vi "rsidr_core_global.vi"() -> ()   [LabVIEW 2020, in "Rohde&Schwarz RTx Oscilloscopes.lvlib"] (continued)
Options"="", "Flags"=0, "Help"="Queries the input capacitance of the probe.\n\nAvailable Repeated Capabilities:\nChannel: CH0, CH1, CH2, CH3, CH4, CHExt\r\n\nRemote-control command(s):\nPROBe<m>:SETup:CAPacitance?"}, {"Level"=2, "Class Only"=FALSE, "Identifier"="RSRTX_ATTR_PROBE_DEGAUSS", "Descriptive Name"="Probe Degauss", "Data Type"=4, "Command"="PROB{Channel}:SET:DEG", "Access"=1, "Range Table"="", "Read Callback"="", "Write Callback"="", "Supported Models"="", "Instrument Options"="", "Flags"=0, "Help"="Demagnetizes the core if it has been magnetized by switching the power on and off, or by an excessive input. Always demagnetize the probe before measurement. The demagnetizing process takes about one second.\n\nAvailable Repeated Capabilities:\nChannel: CH0, CH1, CH2, CH3, CH4, CHExt\r\n\nRemote-control command(s):\nPROBe<m>:SETup:DEGauss"}, {"Level"=2, "Class Only"=FALSE, "Identifier"="RSRTX_ATTR_PROBE_ATTENUATION", "Descriptive Name"="Probe Attenuation", "Data Type"=1, "Command"="PROB{Channel}:SET:ATT?", "Access"=0, "Range Table"="", "Read Callback"="", "Write Callback"="", "Supported Models"="", "Instrument Options"="", "Flags"=0, "Help"="Queries the attenuation of the probe.\n\nAvailable Repeated Capabilities:\nChannel: CH0, CH1, CH2, CH3, CH4, CHExt\r\n\nRemote-control command(s):\nPROBe<m>:SETup:ATTenuation[:AUTO]?"}, {"Level"=2, "Class Only"=FALSE, "Identifier"="RSRTX_ATTR_PROBE_GAIN", "Descriptive Name"="Probe Gain", "Data Type"=1, "Command"="PROB{Channel}:SET:GAIN?", "Access"=0, "Range Table"="RsRtx_rngProbeGain", "Read Callback"="", "Write Callback"="", "Supported Models"="", "Instrument Options"="", "Flags"=0, "Help"="Returns the gain of an automatically detected probe.\n\nAvailable Repeated Capabilities:\nChannel: CH0, CH1, CH2, CH3, CH4, CHExt\r\n\nRemote-control command(s):\nPROBe<m>:SETup:GAIN[:AUTO]?"}, {"Level"=2, "Class Only"=FALSE, "Identifier"="RSRTX_ATTR_PROBE_BANDWIDTH", "Descriptive Name"="Probe Bandwidth", "Data Type"=1, "Command"="PROB{Channel}:SET:BANDwidth?", "Access"=0, "Range Table"="", "Read Callback"="", "Write Callback"="", "Supported Models"="RTM|RTA", "Instrument Options"="", "Flags"=0, "Help"="Queries the bandwidth of the probe.\n\nAvailable Repeated Capabilities:\nChannel: CH0, CH1, CH2, CH3, CH4, CHExt\r\n\nRemote-control command(s):\nPROBe<m>:SETup:BANDwidth?"}, {"Level"=2, "Class Only"=FALSE, "Identifier"="RSRTX_ATTR_PROBE_DC_OFFSET", "Descriptive Name"="Probe DC Offset", "Data Type"=1, "Command"="PROB{Channel}:SET:DCOF?", "Access"=0, "Range Table"="", "Read Callback"="", "Write Callback"="", "Supported Models"="RTM|RTA", "Instrument Options"="", "Flags"=0, "Help"="Retrieves the DC voltage that is measured by the integrated voltmeter of R&S active probes. Switch the voltmeter on before.\n\nAvailable Repeated Capabilities:\nChannel: CH0, CH1, CH2, CH3, CH4, CHExt\r\n\nRemote-control command(s):\nPROBe<m>:SETup:DCOFfset?"}, {"Level"=2, "Class Only"=FALSE, "Identifier"="RSRTX_ATTR_PROBE_CM_OFFSET", "Descriptive Name"="Probe CM Offset", "Data Type"=1, "Command"="PROB{Channel}:SET:CMOF", "Access"=2, "Range Table"="", "Read Callback"="", "Write Callback"="", "Supported Models"="RTM|RTA", "Instrument Options"="", "Flags"=0, "Help"="Configures the CM voltage offset.\n\nAvailable Repeated Capabilities:\nChannel: CH0, CH1, CH2, CH3, CH4, CHExt\r\n\nRemote-control command(s):\nPROBe<m>:SETup:CMOFfset"}, {"Level"=2, "Class Only"=FALSE, "Identifier"="RSRTX_ATTR_PROBE_ADDITIONAL_OFFSET", "Descriptive Name"="Probe Additional Offset", "Data Type"=1, "Command"="PROB{Channel}:SET:UOFF", "Access"=2, "Range Table"="", "Read Callback"="", "Write Callback"="", "Supported Models"="RTM|RTA", "Instrument Options"="", "Flags"=0, "Help"="Sets an additional probe offset.\n\nAvailable Repeated Capabilities:\nChannel: CH0, CH1, CH2, CH3, CH4, CHExt\r\n\nRemote-control command(s):\nPROBe<m>:SETup:UOFFset"}, {"Level"=2, "Class Only"=FALSE, "Identifier"="RSRTX_ATTR_PROBE_VOLTMETER_ENABLED", "Descriptive Name"="Probe Voltmeter Enabled", "Data Type"=3, "Command"="PROB{Channel}:SET:OFFS", "Access"=2, "Range Table"="", "Read Callback"="", "Write Callback"="", "Supported Models"="RTM|RTA", "Instrument Options"="", "Flags"=0, "Help"="Switches the integrated voltmeter of an R&S active probe on or off.\n\nAvailable Repeated Capabilities:\nChannel: CH0, CH1, CH2, CH3, CH4, CHExt\r\n\nRemote-control command(s):\nPROBe<m>:SETup:OFFSwitch"}, {"Level"=2, "Class Only"=FALSE, "Identifier"="RSRTX_ATTR_PROBE_ATTENUATION_UNIT", "Descriptive Name"="Probe Attenuation Unit", "Data Type"=0, "Command"="PROB{Channel}:SET:ATT:UNIT", "Access"=2, "Range Table"="rsrtx_rngProbeUnit", "Read Callback"="", "Write Callback"="", "Supported Models"="", "Instrument Options"="", "Flags"=0, "Help"="Selects the unit that the probe can measure.\n\nAvailable Repeated Capabilities:\nChannel: CH0, CH1, CH2, CH3, CH4, CHExt\r\n\nRemote-control command(s):\nPROBe<m>:SETup:ATTenuation:UNIT"}, {"Level"=2, "Class Only"=FALSE, "Identifier"="RSRTX_ATTR_PROBE_ATTENUATION_MANUAL", "Descriptive Name"="Probe Attenuation Manual", "Data Type"=1, "Command"="PROB{Channel}:SET:ATT:MAN", "Access"=2, "Range Table"="rsrtx_rngProbeAttenuation", "Read Callback"="", "Write Callback"="", "Supported Models"="", "Instrument Options"="", "Flags"=0, "Help"="Sets the attenuation or gain of the probe if the probe was not detected by the instrument.\n\nAvailable Repeated Capabilities:\nChannel: CH0, CH1, CH2, CH3, CH4, CHExt\r\n\nRemote-control command(s):\nPROBe<m>:SETup:ATTenuation:MANual"}, {"Level"=2, "Class Only"=FALSE, "Identifier"="RSRTX_ATTR_PROBE_GAIN_UNIT", "Descriptive Name"="Probe Gain Unit", "Data Type"=0, "Command"="PROB{Channel}:SET:GAIN:UNIT", "Access"=2, "Range Table"="rsrtx_rngProbeUnit", "Read Callback"="", "Write Callback"="", "Supported Models"="", "Instrument Options"="", "Flags"=0, "Help"="Selects the unit that the probe can measure.\n\nAvailable Repeated Capabilities:\nChannel: CH0, CH1, CH2, CH3, CH4, CHExt\r\n\nRemote-control command(s):\nPROBe<m>:SETup:GAIN:UNIT"}, {"Level"=2, "Class Only"=FALSE, "Identifier"="RSRTX_ATTR_PROBE_GAIN_MANUAL", "Descriptive Name"="Probe Gain Manual", "Data Type"=1, "Command"="PROB{Channel}:SET:GAIN:MAN", "Access"=2, "Range Table"="RsRtx_rngProbeGain", "Read Callback"="", "Write Callback"="", "Supported Models"="", "Instrument Options"="", "Flags"=0, "Help"="Sets the gain of the probe. The gain the the reciprocal of the attenuation (RSRTX_ATTR_PROBE_ATTENUATION_MANUAL).\n\nAvailable Repeated Capabilities:\nChannel: CH0, CH1, CH2, CH3, CH4, CHExt\r\n\nRemote-control command(s):\nPROBe<m>:SETup:GAIN:MANual"}, {"Level"=2, "Class Only"=FALSE, "Identifier"="RSRTX_ATTR_PROBE_MICRO_BUTTON_ACTION", "Descriptive Name"="Probe Micro Button Action", "Data Type"=0, "Command"="PROB{Channel}:SET:MODE", "Access"=2, "Range Table"="rsrtx_rngProbeButtonAction", "Read Callback"="", "Write Callback"="", "Supported Models"="RTM|RTA", "Instrument Options"="", "Flags"=0, "Help"="Select the action that is started with the micro button on the probe head.\n\nAvailable Repeated Capabilities:\nChannel: CH0, CH1, CH2, CH3, CH4, CHExt\r\n\nRemote-control command(s):\nPROBe<m>:SETup:MODE"}, {"Level"=2, "Class Only"=FALSE, "Identifier"="RSRTX_ATTR_PROBE_SOFTWARE_VERSION", "Descriptive Name"="Probe Software Version", "Data Type"=2, "Command"="PROB{Channel}:ID:SWV?", "Access"=0, "Range Table"="", "Read Callback"="", "Write Callback"="", "Supported Models"="RTM|RTA", "Instrument Options"="", "Flags"=0, "Help"="Queries the version of the probe firmware.\n\nAvailable Repeated Capabilities:\nChannel: CH0, CH1, CH2, CH3, CH4, CHExt\r\n\nRemote-control command(s):\nPROBe<m>:ID:SWVersion?"}, {"Level"=2, "Class Only"=FALSE, "Identifier"="RSRTX_ATTR_PROBE_PRODUCTION_DATE", "Descriptive Name"="Probe Production Date", "Data Type"=2, "Command"="PROB{Channel}:ID:PRD?", "Access"=0, "Range Table"="", "Read Callback"="", "Write Callback"="", "Supported Models"="RTM|RTA", "Instrument Options"="", "Flags"=0, "Help"="Queries the production date of the probe.\n\nAvailable Repeated Capabilities:\nChannel: CH0, CH1, CH2, CH3, CH4, CHExt\r\n\nRemote-control command(s):\nPROBe<m>:ID:PRDate?"}, {"Level"=2, "Class Only"=FALSE, "Identifier"="RSRTX_ATTR_PROBE_PART_NUMBER", "Descriptive Name"="Probe Part Number", "Data Type"=2, "Command"="PROB{Channel}:ID:PART?", "Access"=0, "Range Table"="", "Read Callback"="", "Write Callback"="", "Supported Models"="RTM|RTA", "Instrument Options"="", "Flags"=0, "Help"="Queries the R&S part number of the probe.\n\nAvailable Repeated Capabilities:\nChannel: CH0, CH1, CH2, CH3, CH4, CHExt\r\n\nRemote-control command(s):\nPROBe<m>:ID:PARTnumber?"}, {"Level"=2, "Class Only"=FALSE, "Identifier"="RSRTX_ATTR_PROBE_BUILD_NUMBER", "Descriptive Name"="Probe Build Number", "Data Type"=0, "Command"="PROB{Channel}:ID:BUIL?", "Access"=0, "Range Table"="", "Read Callback"="", "Write Callback"="", "Supported Models"="RTM|RTA", "Instrument Options"="", "Flags"=0, "Help"="Queries the build number of the probe software.\n\nAvailable Repeated Capabilities:\nChannel: CH0, CH1, CH2, CH3, CH4, CHExt\r\n\nRemote-control command(s):\nPROBe<m>:ID:BUILd?"}, {"Level"=2, "Class Only"=FALSE, "Identifier"="RSRTX_ATTR_PROBE_SERIAL_NUMBER", "Descriptive Name"="Probe Serial Number", "Data Type"=2, "Command"="PROB{Channel}:ID:SRN?", "Access"=0, "Range Table"="", "Read Callback"="", "Write Callback"="", "Supported Models"="RTM|RTA", "Instrument Options"="", "Flags"=0, "Help"="Queries the serial number of the probe.\n\nAvailable Repeated Capabilities:\nChannel: CH0, CH1, CH2, CH3, CH4, CHExt\r\n\nRemote-control command(s):\nPROBe<m>:ID:SRNumber?"}, {"Level"=2, "Class Only"=FALSE, "Identifier"="RSRTX_ATTR_PROBE_COPY_TO_OFFSET", "Descriptive Name"="Probe Copy To Offset", "Data Type"=4, "Command"="PROB{Channel}:SET:ADV:PMT", "Access"=1, "Range Table"="", "Read Callback"="", "Write Callback"="", "Supported Models"="", "Instrument Options"="", "Flags"=0, "Help"="Sets the measured ProbeMeter&apos;s DC mean value as offset. Make sure that the Probe-Meter is active before you use this attribute.\n\nAvailable Repeated Capabilities:\nChannel: CH0, CH1, CH2, CH3, CH4, CHExt\r\n\nRemote-control command(s):\nPROBe<m>:SETup:ADVanced:PMToffset"}, {"Level"=2, "Class Only"=FALSE, "Identifier"="RSRTX_ATTR_PROBE_ATTENUATOR_RT_ZA15_ENABLED", "Descriptive Name"="Probe Attenuator RT ZA15 Enabled", "Data Type"=3, "Command"="PROB{Channel}:SET:ZAXV", "Access"=2, "Range Table"="", "Read Callback"="", "Write Callback"="", "Supported Models"="", "Instrument Options"="", "Flags"=0, "Help"="Relevant only for differential active probes R&S RT-ZD10, R&S RT-ZD20 or R&S RT-ZD30. If you use the external attenuator R&S RT-ZA15, enable it to include the external attenuation in the measurements.\n\nAvailable Repeated Capabilities:\nChannel: CH0, CH1, CH2, CH3, CH4, CHExt\r\n\nRemote-control command(s):\nPROBe<m>:SETup:ZAXV"}, {"Level"=2, "Class Only"=FALSE, "Identifier"="RSRTX_ATTR_PROBE_ZERO_ADJUST", "Descriptive Name"="Probe Zero Adjust", "Data Type"=1, "Command"="PROB{Channel}:SET:ADV:ZADJ", "Access"=2, "Range Table"="RsRtx_rngProbeZeroAdjust", "Read Callback"="", "Write Callback"="", "Supported Models"="", "Instrument Options"="", "Flags"=0, "Help"="Relevant only for R&S RT-ZCxxB current probes. It sets the waveform to zero position. It corrects the effect of a voltage offset or temperature drift.\n\nAvailable Repeated Capabilities:\nChannel: CH0, CH1, CH2, CH3, CH4, CHExt\r\n\nRemote-control command(s):\nPROBe<m>:SETup:ADVanced:ZADJust"}, {"Level"=2, "Class Only"=FALSE, "Identifier"="RSRTX_ATTR_PROBE_SAVE_ZERO_ADJUST", "Descriptive Name"="Probe Save Zero Adjust", "Data Type"=4, "Command"="PROB{Channel}:SET:ADV:STPR", "Access"=1, "Range Table"="", "Read Callback"="", "Write Callback"="", "Supported Models"="", "Instrument Options"="", "Flags"=0, "Help"="Relevant only for R&S RT-ZCxxB current probes. It saves the zero adjust value in the probe box. If you connect the probe to another channel or to another oscilloscope with Rohde & Schwarz probe interface, the value is read out again.\n\nAvailable Repeated Capabilities:\nChannel: CH0, CH1, CH2, CH3, CH4, CHExt\r\n\nRemote-control command(s):\nPROBe<m>:SETup:ADVanced:STPRobe"}, {"Level"=2, "Class Only"=FALSE, "Identifier"="RSRTX_ATTR_PROBE_INPUT_VOLTAGE_RANGE", "Descriptive Name"="Probe Input Voltage Range", "Data Type"=0, "Command"="PROB{Channel}:SET:ADV:RANG", "Access"=2, "Range Table"="RsRtx_rngProbeInputVoltageRange", "Read Callback"="", "Write Callback"="", "Supported Models"="", "Instrument Options"="", "Flags"=0, "Help"="Relevant for R&S RT-ZHD probes. It sets the voltage range of the probe.\n\nAvailable Repeated Capabilities:\nChannel: CH0, CH1, CH2, CH3, CH4, CHExt\r\n\nRemote-control command(s):\nPROBe<m>:SETup:ADVanced:RANGe"}, {"Level"=2, "Class Only"=FALSE, "Identifier"="RSRTX_ATTR_PROBE_BANDWIDTH_LIMIT", "Descriptive Name"="Probe Bandwidth Limit", "Data Type"=3, "Command"="PROB{Channel}:SET:ADV:FILT", "Access"=2, "Range Table"="", "Read Callback"="", "Write Callback"="", "Supported Models"="", "Instrument Options"="", "Flags"=0, "Help"="Relevant for R&S RT-ZHD probes. It activates the lowpass filter in the probe control box.\n\nAvailable Repeated Capabilities:\nChannel: CH0, CH1, CH2, CH3, CH4, CHExt\r\n\nRemote-control command(s):\nPROBe<m>:SETup:ADVanced:FILTer"}, {"Level"=2, "Class Only"=FALSE, "Identifier"="RSRTX_ATTR_PROBE_AUDIBLE_OVERRANGE", "Descriptive Name"="Probe Audible Overrange", "Data Type"=3, "Command"="PROB{Channel}:SET:ADV:AUD", "Access"=2, "Range Table"="", "Read Callback"="", "Write Callback"="", "Supported Models"="", "Instrument Options"="", "Flags"=0, "Help"="Relevant for R&S RT-ZHD probes. It activates the acoustic overrange warning in the probe control box.\n\nAvailable Repeated Capabilities:\nChannel: CH0, CH1, CH2, CH3, CH4, CHExt\r\n\nRemote-control command(s):\nPROBe<m>:SETup:ADVanced:AUDioverload"}, {"Level"=2, "Class Only"=FALSE, "Identifier"="RSRTX_ATTR_PROBE_MEAS_MODE", "Descriptive Name"="Probe Meas Mode", "Data Type"=0, "Command"="PROB{Channel}:SET:PRM", "Access"=2, "Range Table"="RsRtx_rngProbeMeasMode", "Read Callback"="", "Write Callback"="", "Supported Models"="", "Instrument Options"="", "Flags"=0, "Help"="Relevant only for R&S RT-ZM probes. It sets the measurement mode of modular probes. You can switch between singleended, differential and common mode measurements without reconnecting or resoldering the probe.\n\nAvailable Repeated Capabilities:\nChannel: CH0, CH1, CH2, CH3, CH4, CHExt\r\n\nRemote-control command(s):\nPROBe<m>:SETup:PRMode"}, {"Level"=2, "Class Only"=FALSE, "Identifier"="RSRTX_ATTR_PROBE_AC_COUPLING", "Descriptive Name"="Probe AC Coupling", "Data Type"=3, "Command"="PROB{Channel}:SET:ACC", "Access"=2, "Range Table"="", "Read Callback"="", "Write Callback"="", "Supported Models"="", "Instrument Options"="", "Flags"=0, "Help"="Enables AC coupling in R&S RT-ZPR probes, which removes DC and very low-frequency components. The R&S RT-ZPR probes requires 50   input termination, for which the channel AC coupling is not available. The probe setting allows AC coupling also at 50   inputs.\n\nAvailable Repeated Capabilities:\nChannel: CH0, CH1, CH2, CH3, CH4, CHExt\r\n\nRemote-control command(s):\nPROBe<m>:SETup:ACCoupling"}, {"Level"=2, "Class Only"=TRUE, "Identifier"="", "Descriptive Name"="Probe Meter", "Data Type"=0, "Command"="", "Access"=0, "Range Table"="", "Read Callback"="", "Write Callback"="", "Supported Models"="", "Instrument Options"="", "Flags"=0, "Help"="Shows the measurement result of the integrated R&S ProbeMeter of active Rohde & Schwarz voltage probes.\nIf a single-ended or power rail probe is connected, the ProbeMeter measures DC voltages between the probe tip and ground connection and enables ground-referenced measurements of voltages.\nIf a differential probe is connected, the ProbeMeter measures differential and common\nmode voltages.\nThe ProbeMeter measures continuously and in parallel to the measurements of the oscilloscope. The results are shown below the grid. You can switch off the ProbeMeter using the button below the the results."}, {"Level"=3, "Class Only"=FALSE, "Identifier"="RSRTX_ATTR_PROBE_METER_VISIBILITY", "Descriptive Name"="Probe Meter Visibility", "Data Type"=3, "Command"="PROB{Channel}:PMET:VIS", "Access"=2, "Range Table"="", "Read Callback"="", "Write Callback"="", "Supported Models"="", "Instrument Options"="", "Flags"=0, "Help"="Switches the integrated voltmeter of a Rohde & Schwarz active probe on or off. Only relevant if a Rohde & Schwarz active probe with R&S ProbeMeter is used.\n\nAvailable Repeated Capabilities:\nChannel: CH0, CH1, CH2, CH3, CH4, CHExt\r\n\nRemote-control command(s):\nPROBe<m>:PMETer:VISibility"}, {"Level"=3, "Class Only"=FALSE, "Identifier"="RSRTX_ATTR_PROBE_METER_RESULT_SINGLE", "Descriptive Name"="Probe Meter Result Single", "Data Type"=1, "Command"="PROB{Channel}:PMET:RES:SING?", "Access"=0, "Range Table"="", "Read Callback"="", "Write Callback"="", "Supported Models"="", "Instrument Options"="", "Flags"=0, "Help"="Returns probe meter single result.\n\nAvailable Repeated Capabilities:\nChannel: CH0, CH1, CH2, CH3, CH4, CHExt\r\n\nRemote-control command(s):\nPROBe<m>:PMETer:RESults:SINGle?"}, {"Level"=3, "Class Only"=FALSE, "Identifier"="RSRTX_ATTR_PROBE_METER_RESULT_COMMON", "Descriptive Name"="Probe Meter Result Common", "Data Type"=1, "Command"="PROB{Channel}:PMET:RES:COMM?", "Access"=0, "Range Table"="", "Read Callback"="", "Write Callback"="", "Supported Models"="", "Instrument Options"="", "Flags"=0, "Help"="It returns the common mode voltage, which is the mean voltage between the signal sockets and the ground socket.\n\nAvailable Repeated Capabilities:\nChannel: CH0, CH1, CH2, CH3, CH4, CHExt\r\n\nRemote-control command(s):\nPROBe<m>:PMETer:RESults:COMMon?"}, {"Level"=3, "Class Only"=FALSE, "Identifier"="RSRTX_ATTR_PROBE_METER_RESULT_DIFFERENTIAL", "Descriptive Name"="Probe Meter Result Differential", "Data Type"=1, "Command"="PROB{Channel}:PMET:RES:DIFF?", "Access"=0, "Range Table"="", "Read Callback"="", "Write Callback"="", "Supported Models"="", "Instrument Options"="", "Flags"=0, "Help"="It returns the differential voltage, which is the voltage between the positive and negative signal sockets.\n\nAvailable Repeated Capabilities:\nChannel: CH0, CH1, CH2, CH3, CH4, CHExt\r\n\nRemote-control command(s):\nPROBe<m>:PMETer:RESults:DIFFerential?"}, {"Level"=3, "Class Only"=FALSE, "Identifier"="RSRTX_ATTR_PROBE_METER_RESULT_NEGATIVE", "Descriptive Name"="Probe Meter Result Negative", "Data Type"=1, "Command"="PROB{Channel}:PMET:RES:NEG?", "Access"=0, "Range Table"="", "Read Callback"="", "Write Callback"="", "Supported Models"="", "Instrument Options"="", "Flags"=0, "Help"="It returns the voltage that is measured between the negative signal socket and the ground.\n\nAvailable Repeated Capabilities:\nChannel: CH0, CH1, CH2, CH3, CH4, CHExt\r\n\nRemote-control command(s):\nPROBe<m>:PMETer:RESults:NEGative?"}, {"Level"=3, "Class Only"=FALSE, "Identifier"="RSRTX_ATTR_PROBE_METER_RESULT_POSITIVE", "Descriptive Name"="Probe Meter Result Positive", "Data Type"=1, "Command"="PROB{Channel}:PMET:RES:POS?", "Access"=0, "Range Table"="", "Read Callback"="", "Write Callback"="", "Supported Models"="", "Instrument Options"="", "Flags"=0, "Help"="It returns the voltage that is measured between the positive signal socket and the ground.\n\nAvailable Repeated Capabilities:\nChannel: CH0, CH1, CH2, CH3, CH4, CHExt\r\n\nRemote-control command(s):\nPROBe<m>:PMETer:RESults:POSitive?"}, {"Level"=1, "Class Only"=TRUE, "Identifier"="", "Descriptive Name"="Label", "Data Type"=0, "Command"="", "Access"=0, "Range Table"="", "Read Callback"="", "Write Callback"="", "Supported Models"="", "Instrument Options"="", "Flags"=0, "Help"="The class contains attributes where you can define an additional name label for the selected waveform."}, {"Level"=2, "Class Only"=FALSE, "Identifier"="RSRTX_ATTR_LABEL_ENABLED", "Descriptive Name"="Label Enabled", "Data Type"=3, "Command"="CHAN{Channel}:LAB:STAT", "Access"=2, "Range Table"="", "Read Callback"="", "Write Callback"="", "Supported Models"="", "Instrument Options"="", "Flags"=0, "Help"="Switches the channel name on or off.\n\nAvailable Repeated Capabilities:\nChannel: CH0, CH1, CH2, CH3, CH4, CHExt\r\n\nRemote-control command(s):\nCHANnel<ml>:LABel:STATe"}, {"Level"=2, "Class Only"=FALSE, "Identifier"="RSRTX_ATTR_LABEL_NAME", "Descriptive Name"="Label Name", "Data Type"=2, "Command"="CHAN{Channel}:LAB", "Access"=2, "Range Table"="", "Read Callback"="", "Write Callback"="", "Supported Models"="", "Instrument Options"="", "Flags"=0, "Help"="Specifies a name for the selected channel.\n\nAvailable Repeated Capabilities:\nChannel: CH0, CH1, CH2, CH3, CH4, CHExt\r\n\nRemote-control command(s):\nCHANnel<m>:LABel"}, {"Level"=2, "Class Only"=TRUE, "Identifier"="", "Descriptive Name"="Bus", "Data Type"=0, "Command"="", "Access"=0, "Range Table"="", "Read Callback"="", "Write Callback"="", "Supported Models"="", "Instrument Options"="", "Flags"=0, "Help"="Contain attributes for settings of Bus Label."}, {"Level"=3, "Class Only"=FALSE, "Identifier"="RSRTX_ATTR_BUS_LABEL_ENABLED", "Descriptive Name"="Bus Label Enabled", "Data Type"=3, "Command"="BUS{SerialBus}:LAB:STAT", "Access"=2, "Range Table"="", "Read Callback"="", "Write Callback"="", "Supported Models"="", "Instrument Options"="", "Flags"=0, "Help"="Displays or hides the bus label. The bus label is shown on the the right side of the display.\n\nAvailable Repeated Capabilities:\nSerialBus: SB1, SB2, SB3, SB4\r\n\nRemote-control command(s):\nBUS<b>:LABel:STATe"}, {"Level"=3, "Class Only"=FALSE, "Identifier"="RSRTX_ATTR_BUS_LABEL_NAME", "Descriptive Name"="Bus Label Name", "Data Type"=2, "Command"="BUS{SerialBus}:LAB", "Access"=2, "Range Table"="", "Read Callback"="", "Write Callback"="", "Supported Models"="", "Instrument Options"="", "Flags"=0, "Help"="Defines an additional name label for the selected bus. The maximum name length is 8 characters, and only ASCII characters can be used.\n\nAvailable Repeated Capabilities:\nSerialBus: SB1, SB2, SB3, SB4\r\n\nRemote-control command(s):\nBUS<b>:LABel"}, {"Level"=1, "Class Only"=TRUE, "Identifier"="", "Descriptive Name"="Channel Subsystem", "Data Type"=0, "Command"="", "Access"=0, "Range Table"="", "Read Callback"="", "Write Callback"="", "Supported Models"="", "Instrument Options"="", "Flags"=0, "Help"="Channel-based attributes that you use to configure the channel subsystemof the oscilloscope.  All of the channel subsystem attributes are channel-based."}, {"Level"=2, "Class Only"=FALSE, "Identifier"="RSRTX_ATTR_CHANNEL_ENABLED", "Descriptive Name"="Channel Enabled", "Data Type"=3, "Command"="CHAN{Channel}:STAT", "Access"=2, "Range Table"="", "Read Callback"="", "Write Callback"="", "Supported Models"="", "Instrument Options"="", "Flags"=0, "Help"="Switches the channel signal on or off.\n\nAvailable Repeated Capabilities:\nChannel: CH0, CH1, CH2, CH3, CH4, CHExt\r\n\nRemote-control command(s):\nCHANnel<m>:STATe"}, {"Level"=2, "Class Only"=FALSE, "Identifier"="RSRTX_ATTR_VERTICAL_RANGE", "Descriptive Name"="Vertical Range", "Data Type"=1, "Command"="CHAN{Channel}:RANG", "Access"=2, "Range Table"="", "Read Callback"="", "Write Callback"="", "Supported Models"="", "Instrument Options"="", "Flags"=0, "Help"="Sets the voltage range across the 10 vertical divisions of the diagram.\n\nAvailable Repeated Capabilities:\nChannel: CH0, CH1, CH2, CH3, CH4, CHExt\r\n\nRemote-control command(s):\nCHANnel<m>:RANGe"}, {"Level"=2, "Class Only"=FALSE, "Identifier"="RSRTX_ATTR_VERTICAL_COUPLING", "Descriptive Name"="Vertical Coupling", "Data Type"=0, "Command"="CHAN{Channel}:COUP", "Access"=2, "Range Table"="rsrtx_rngVerticalCoupling", "Read Callback"="", "Write Callback"="", "Supported Models"="", "Instrument Options"="", "Flags"=0, "Help"="Selects the connection of the indicated channel signal.\n\nAvailable Repeated Capabilities:\nChannel: CH0, CH1, CH2, CH3, CH4, CHExt\r\n\nRemote-control command(s):\nCHANnel<m>:COUPling"}, {"Level"=2, "Class Only"=FALSE, "Identifier"="RSRTX_ATTR_VERTICAL_SCALE", "Descriptive Name"="Vertical Scale", "Data Type"=1, "Command"="CHAN{Channel}:SCAL", "Access"=2, "Range Table"="", "Read Callback"="", "Write Callback"="", "Supported Models"="", "Instrument Options"="", "Flags"=0, "Help"="Sets the vertical range per division.\n\nAvailable Repeated Capabilities:\nChannel: CH0, CH1, CH2, CH3, CH4, CHExt\r\n\nRemote-control command(s):\nCHANnel<m>:SCALe"}, {"Level"=2, "Class Only"=FALSE, "Identifier"="RSRTX_ATTR_CHANNEL_OFFSET", "Descriptive Name"="Channel Offset", "Data Type"=1, "Command"="CHAN{Channel}:OFFS", "Access"=2, "Range Table"="", "Read Callback"="", "Write Callback"="", "Supported Models"="", "Instrument Options"="", "Flags"=0, "Help"="The offset voltage is subtracted to correct an offset-affected signal.\n\nAvailable Repeated Capabilities:\nChannel: CH0, CH1, CH2, CH3, CH4, CHExt\r\n\nRemote-control command(s):\nCHANnel<m>:OFFSet"}, {"Level"=2, "Class Only"=FALSE, "Identifier"="RSRTX_ATTR_CHANNEL_ZERO_OFFSET", "Descriptive Name"="Channel Zero Offset", "Data Type"=1, "Command"="CHAN{Channel}:ZOFF", "Access"=2, "Range Table"="", "Read Callback"="", "Write Callback"="", "Supported Models"="", "Instrument Options"="", "Flags"=0, "Help"="Sets the zero offset. Differences in DUT and oscilloscope ground levels may cause larger zero errors affecting the waveform. If the DUT is ground-referenced, the Zero Offset corrects the zero error and sets the probe to the zero level. You can assess the zero error by measuring the mean value of a signal that should return zero.\n\nAvailable Repeated Capabilities:\nChannel: CH0, CH1, CH2, CH3, CH4, CHExt\r\n\nRemote-control command(s):\nCHANnel<m>:ZOFFset[:VALue]"}, {"Level"=2, "Class Only"=FALSE, "Identifier"="RSRTX_ATTR_CHANNEL_BANDWIDTH_LIMIT", "Descriptive Name"="Channel Bandwidth Limit", "Data Type"=0, "Command"="CHAN{Channel}:BAND", "Access"=2, "Range Table"="rsrtx_rngChannelBWLimit", "Read Callback"="", "Write Callback"="", "Supported Models"="", "Instrument Options"="", "Flags"=0, "Help"="Selects the bandwidth limit for the indicated channel.\n\nAvailable Repeated Capabilities:\nChannel: CH0, CH1, CH2, CH3, CH4, CHExt\r\n\nRemote-control command(s):\nCHANnel<m>:BANDwidth"}, {"Level"=2, "Class Only"=FALSE, "Identifier"="RSRTX_ATTR_CHANNEL_POLARITY", "Descriptive Name"="Channel Polarity", "Data Type"=0, "Command"="CHAN{Channel}:POL", "Access"=2, "Range Table"="rsrtx_rngChannelPolarity", "Read Callback"="", "Write Callback"="", "Supported Models"="", "Instrument Options"="", "Flags"=0, "Help"="Turns the inversion of the signal amplitude on or off. To invert means to reflect the voltage values of all signal components against the ground level. Inversion affects only the display of the signal but not the trigger.\n\nAvailable Repeated Capabilities:\nChannel: CH0, CH1, CH2, CH3, CH4, CHExt\r\n\nRemote-control command(s):\nCHANnel<m>:POLarity"}, {"Level"=2, "Class Only"=FALSE, "Identifier"="RSRTX_ATTR_CHANNEL_OVERLOAD", "Descriptive Name"="Channel Overload", "Data Type"=3, "Command"="CHAN{Channel}:OVER", "Access"=2, "Range Table"="", "Read Callback"="", "Write Callback"="", "Supported Models"="", "Instrument Options"="", "Flags"=0, "Help"="Retrieves the overload status of the specified channel from the status bit. When the overload problem is solved, the command resets the status bit. Use VI_FALSE to clear the overload condition.\n\nAvailable Repeated Capabilities:\nChannel: CH0, CH1, CH2, CH3, CH4, CHExt\r\n\nRemote-control command(s):\nCHANnel<m>:OVERload"}, {"Level"=2, "Class Only"=FALSE, "Identifier"="RSRTX_ATTR_CHANNEL_SKEW", "Descriptive Name"="Channel Skew", "Data Type"=1, "Command"="CHAN{Channel}:SKEW", "Access"=2, "Range Table"="", "Read Callback"="", "Write Callback"="", "Supported Models"="", "Instrument Options"="", "Flags"=0, "Help"="Skew or deskew compensates delay differences between channels caused by the different length of cables, probes, and other sources. Correct deskew values are important for accurate triggering.\n\nAvailable Repeated Capabilities:\nChannel: CH0, CH1, CH2, CH3, CH4, CHExt\r\n\nRemote-control command(s):\nCHANnel<m>:SKEW"}, {"Level"=2, "Class Only"=FALSE, "Identifier"="RSRTX_ATTR_CHANNEL_THRESHOLD", "Descriptive Name"="Channel Threshold", "Data Type"=1, "Command"="CHAN{Channel}:THR", "Access"=2, "Range Table"="", "Read Callback"="", "Write Callback"="", "Supported Models"="", "Instrument Options"="", "Flags"=0, "Help"="Threshold value for digitization of analog signals. If the signal value is higher than the threshold, the signal state is high (1 or true for the boolean logic). Otherwise, the signal state is considered low (0 or false) if the signal value is below the threshold.\n\nAvailable Repeated Capabilities:\nChannel: CH0, CH1, CH2, CH3, CH4, CHExt\r\n\nRemote-control command(s):\nCHANnel<m>:THReshold"}, {"Level"=2, "Class Only"=FALSE, "Identifier"="RSRTX_ATTR_CHANNEL_THRESHOLD_HYSTERESIS", "Descriptive Name"="Channel Threshold Hysteresis", "Data Type"=0, "Command"="CHAN{Channel}:THR:HYST", "Access"=2, "Range Table"="rsrtx_rngThresholdHysteresis", "Read Callback"="", "Write Callback"="", "Supported Models"="", "Instrument Options"="", "Flags"=0, "Help"="Defines the size of the hysteresis to avoid the change of signal states due to noise.\n\nAvailable Repeated Capabilities:\nChannel: CH0, CH1, CH2, CH3, CH4, CHExt\r\n\nRemote-control command(s):\nCHANnel<m>:THReshold:HYSTeresis"}, {"Level"=2, "Class Only"=FALSE, "Identifier"="RSRTX_ATTR_CHANNEL_POSITION", "Descriptive Name"="Channel Position", "Data Type"=1, "Command"="CHAN{Channel}:POS", "Access"=2, "Range Table"="RsRtx_rngChannelPosition", "Read Callback"="", "Write Callback"="", "Supported Models"="", "Instrument Options"="", "Flags"=0, "Help"="Sets the vertical position of the waveform in divisions. While the offset sets a voltage, position is a graphical setting given in divisions.\n\nAvailable Repeated Capabilities:\nChannel: CH0, CH1, CH2, CH3, CH4, CHExt\r\n\nRemote-control command(s):\nCHANnel<m>:POSition"}, {"Level"=2, "Class Only"=FALSE, "Identifier"="RSRTX_ATTR_CHANNEL_WAVEFORM_COLOR", "Descriptive Name"="Channel Waveform Color", "Data Type"=0, "Command"="CHAN{Channel}:WCOL", "Access"=2, "Range Table"="RsRtx_rngChannelWaveformColor", "Read Callback"="", "Write Callback"="", "Supported Models"="", "Instrument Options"="", "Flags"=0, "Help"="Selects the color scale for the waveform color. Each scale comprises a set of colors, where each color represents a certain frequency of occurrence.\n\nAvailable Repeated Capabilities:\nChannel: CH0, CH1, CH2, CH3, CH4, CHExt\r\n\nRemote-control command(s):\nCHANnel<m>:WCOLor"}, {"Level"=2, "Class Only"=FALSE, "Identifier"="RSRTX_ATTR_PROTOCOL_FIND_LEVEL", "Descriptive Name"="Protocol Find Level", "Data Type"=4, "Command"="CHAN{Channel}:THR:FIND", "Access"=1, "Range Table"="", "Read Callback"="", "Write Callback"="", "Supported Models"="", "Instrument Options"="", "Flags"=0, "Help"="Executes the analysis of all channels that are configured for the selected bus and sets the threshold for digitization of analog signals for each channel\n\nAvailable Repeated Capabilities:\nChannel: CH0, CH1, CH2, CH3, CH4, CHExt\r\n\nRemote-control command(s):\nCHANnel<m>:THReshold:FINDlevel"}, {"Level"=2, "Class Only"=FALSE, "Identifier"="RSRTX_ATTR_CHANNEL_ALL_OFF", "Descriptive Name"="Channel All Off", "Data Type"=4, "Command"="CHAN:AOFF", "Access"=1, "Range Table"="", "Read Callback"="", "Write Callback"="", "Supported Models"="", "Instrument Options"="", "Flags"=0, "Help"="Switches all analog channels off.\n\nAvailable Repeated Capabilities:\nNone\n\nRemote-control command(s):\nCHANnel<m>:AOFF"}, {"Level"=2, "Class Only"=FALSE, "Identifier"="RSRTX_ATTR_CHANNEL_ALL_ON", "Descriptive Name"="Channel All On", "Data Type"=4, "Command"="CHAN:AON", "Access"=1, "Range Table"="", "Read Callback"="", "Write Callback"="", "Supported Models"="", "Instrument Options"="", "Flags"=0, "Help"="Switches all analog channels on.\n\nAvailable Repeated Capabilities:\nNone\n\nRemote-control command(s):\nCHANnel<m>:AON"}, {"Level"=1, "Class Only"=TRUE, "Identifier"="", "Descriptive Name"="Digital Channel", "Data Type"=0, "Command"="", "Access"=0, "Range Table"="", "Read Callback"="", "Write Callback"="", "Supported Models"="", "Instrument Options"="", "Flags"=0, "Help"="Digital settings."}, {"Level"=2, "Class Only"=FALSE, "Identifier"="RSRTX_ATTR_DIGITAL_ENABLED", "Descriptive Name"="Digital Enabled", "Data Type"=3, "Command"="DIG{Digital}:DISP", "Access"=2, "Range Table"="", "Read Callback"="", "Write Callback"="", "Supported Models"="", "Instrument Options"="", "Flags"=0, "Help"="Enables and displays the indicated digital channel, or disables it.\n\nAvailable Repeated Capabilities:\nDigital: D0, D1, D2, D3, D4, D5, D6, D7, D8, D9, D10, D11, D12, D13, D14, D15\r\n\nRemote-control command(s):\nDIGital<m>:DISPlay"}, {"Level"=2, "Class Only"=FALSE, "Identifier"="RSRTX_ATTR_DIGITAL_DESKEW", "Descriptive Name"="Digital Deskew", "Data Type"=1, "Command"="DIG{Digital}:DESK", "Access"=2, "Range Table"="", "Read Callback"="", "Write Callback"="", "Supported Models"="RTM|RTA", "Instrument Options"="", "Flags"=0, "Help"="Sets the deskew values, one value for each pod. The deskew value compensates\ndelays that are known from the circuit specifics or caused by the different length of\ncables. The skew between the probe boxes of the digital channels and the probe con-\nnectors of the analog channels is automatically aligned by the instrument.\n\nAvailable Repeated Capabilities:\nDigital: D0, D1, D2, D3, D4, D5, D6, D7, D8, D9, D10, D11, D12, D13, D14, D15\r\n\nRemote-control command(s):\nDIGital<m>:DESKew"}, {"Level"=2, "Class Only"=FALSE, "Identifier"="RSRTX_ATTR_DIGITAL_THRESHOLD", "Descriptive Name"="Digital Threshold", "Data Type"=1, "Command"="DIG{Digital}:THR", "Access"=2, "Range Table"="", "Read Callback"="", "Write Callback"="", "Supported Models"="", "Instrument Options"="", "Flags"=0, "Help"="Sets the logical threshold for the channel group to which the indicated digital channel belongs.\n\nAvailable Repeated Capabilities:\nDigital: D0, D1, D2, D3, D4, D5, D6, D7, D8, D9, D10, D11, D12, D13, D14, D15\r\n\nRemote-control command(s):\nDIGital<m>:THReshold"}, {"Level"=2, "Class Only"=FALSE, "Identifier"="RSRTX_ATTR_DIGITAL_TECHNOLOGY", "Descriptive Name"="Digital Technology", "Data Type"=0, "Command"="DIG{Digital}:TECH", "Access"=2, "Range Table"="rsrtx_rngDigitalTechnology", "Read Callback"="", "Write Callback"="", "Supported Models"="", "Instrument Options"="", "Flags"=0, "Help"="Selects the threshold voltage for various types of integrated circuits and applies it to the channel group to which the indicated digital channel belongs.\n\nAvailable Repeated Capabilities:\nDigital: D0, D1, D2, D3, D4, D5, D6, D7, D8, D9, D10, D11, D12, D13, D14, D15\r\n\nRemote-control command(s):\nDIGital<m>:TECHnology"}, {"Level"=2, "Class Only"=FALSE, "Identifier"="RSRTX_ATTR_DIGITAL_HYSTERESIS", "Descriptive Name"="Digital Hysteresis", "Data Type"=0, "Command"="DIG{Digital}:HYST", "Access"=2, "Range Table"="rsrtx_rngDigitalHysteresis", "Read Callback"="", "Write Callback"="", "Supported Models"="", "Instrument Options"="", "Flags"=0, "Help"="Defines the size of the hysteresis to avoid the change of signal states due to noise. The setting applied to the channel group to which the indicated digital channel belongs.\n\nAvailable Repeated Capabilities:\nDigital: D0, D1, D2, D3, D4, D5, D6, D7, D8, D9, D10, D11, D12, D13, D14, D15\r\n\nRemote-control command(s):\nDIGital<m>:HYSTeresis"}, {"Level"=2, "Class Only"=FALSE, "Identifier"="RSRTX_ATTR_DIGITAL_APPLY", "Descriptive Name"="Digital Apply", "Data Type"=3, "Command"="DIG:THC", "Access"=2, "Range Table"="", "Read Callback"="", "Write Callback"="", "Supported Models"="RTM|RTA", "Instrument Options"="", "Flags"=0, "Help"="Sets all threshold and hysteresis values to the values of the first nibble (D0...D3).\n\nAvailable Repeated Capabilities:\nNone\n\nRemote-control command(s):\nDIGital<m>:THCoupling"}, {"Level"=2, "Class Only"=FALSE, "Identifier"="RSRTX_ATTR_DIGITAL_LABEL", "Descriptive Name"="Digital Label", "Data Type"=2, "Command"="DIG{Digital}:LAB", "Access"=2, "Range Table"="", "Read Callback"="", "Write Callback"="", "Supported Models"="", "Instrument Options"="", "Flags"=0, "Help"="Defines a label for the indicated digital channel.\n\nAvailable Repeated Capabilities:\nDigital: D0, D1, D2, D3, D4, D5, D6, D7, D8, D9, D10, D11, D12, D13, D14, D15\r\n\nRemote-control command(s):\nDIGital<m>:LABel"}, {"Level"=2, "Class Only"=FALSE, "Identifier"="RSRTX_ATTR_DIGITAL_LABEL_ENABLED", "Descriptive Name"="Digital Label Enabled", "Data Type"=3, "Command"="DIG{Digital}:LAB:STAT", "Access"=2, "Range Table"="", "Read Callback"="", "Write Callback"="", "Supported Models"="", "Instrument Options"="", "Flags"=0, "Help"="Displays or hides the label of the indicated digital channel.\n\nAvailable Repeated Capabilities:\nDigital: D0, D1, D2, D3, D4, D5, D6, D7, D8, D9, D10, D11, D12, D13, D14, D15\r\n\nRemote-control command(s):\nDIGital<m>:LABel:STATe"}, {"Level"=2, "Class Only"=FALSE, "Identifier"="RSRTX_ATTR_DIGITAL_VERTICAL_CHANNEL_SIZE", "Descriptive Name"="Digital Vertical Channel Size", "Data Type"=1, "Command"="DIG{Digital}:SIZE", "Access"=2, "Range Table"="", "Read Callback"="", "Write Callback"="", "Supported Models"="", "Instrument Options"="", "Flags"=0, "Help"="Sets the size of the indicated vertical channel.\n\nAvailable Repeated Capabilities:\nDigital: D0, D1, D2, D3, D4, D5, D6, D7, D8, D9, D10, D11, D12, D13, D14, D15\r\n\nRemote-control command(s):\nDIGital<m>:SIZE"}, {"Level"=2, "Class Only"=FALSE, "Identifier"="RSRTX_ATTR_DIGITAL_VERTICAL_POSITION", "Descriptive Name"="Digital Vertical Position", "Data Type"=1, "Command"="DIG{Digital}:POS", "Access"=2, "Range Table"="", "Read Callback"="", "Write Callback"="", "Supported Models"="", "Instrument Options"="", "Flags"=0, "Help"="Sets the vertical position of the indicated vertical channel.\n\nAvailable Repeated Capabilities:\nDigital: D0, D1, D2, D3, D4, D5, D6, D7, D8, D9, D10, D11, D12, D13, D14, D15\r\n\nRemote-control command(s):\nDIGital<m>:POSition"}, {"Level"=2, "Class Only"=FALSE, "Identifier"="RSRTX_ATTR_DIGITAL_CURRENT_STATUS_MAXIMUM", "Descriptive Name"="Digital Current Status Maximum", "Data Type"=3, "Command"="DIG{Digital}:CURR:STAT:MAX?", "Access"=0, "Range Table"="", "Read Callback"="", "Write Callback"="", "Supported Models"="", "Instrument Options"="", "Flags"=0, "Help"="Returns the current status maximum of the indicated digital channel regardless of the trigger settings, and even without any acquisition.\n\nAvailable Repeated Capabilities:\nDigital: D0, D1, D2, D3, D4, D5, D6, D7, D8, D9, D10, D11, D12, D13, D14, D15\r\n\nRemote-control command(s):\nDIGital<m>:CURRent:STATe:MAXimum?"}, {"Level"=2, "Class Only"=FALSE, "Identifier"="RSRTX_ATTR_DIGITAL_CURRENT_STATUS_MINIMUM", "Descriptive Name"="Digital Current Status Minimum", "Data Type"=3, "Command"="DIG{Digital}:CURR:STAT:MIN?", "Access"=0, "Range Table"="", "Read Callback"="", "Write Callback"="", "Supported Models"="", "Instrument Options"="", "Flags"=0, "Help"="Returns the current status minimum of the indicated digital channel regardless of the trigger settings, and even without any acquisition.\n\nAvailable Repeated Capabilities:\nDigital: D0, D1, D2, D3, D4, D5, D6, D7, D8, D9, D10, D11, D12, D13, D14, D15\r\n\nRemote-control command(s):\nDIGital<m>:CURRent:STATe:MINimum?"}, {"Level"=2, "Class Only"=FALSE, "Identifier"="RSRTX_ATTR_DIGITAL_PROBE_ENABLED", "Descriptive Name"="Digital Probe Enabled", "Data Type"=3, "Command"="DIG{Digital}:PROB:ENAB?", "Access"=0, "Range Table"="", "Read Callback"="", "Write Callback"="", "Supported Models"="", "Instrument 
